vi "Thread@ElseIf__Parameter.vi"(1 "ParamterIn":string) -> (0 "ParamterOut":string)   [LabVIEW 2020]
panel:
  in  "Logic":string(combo)
  in  "Confirm":bool
  # "Thread@ElseIf $Logic"
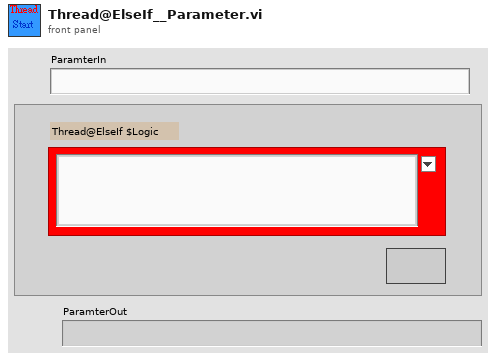
[diagram p1: front panel]
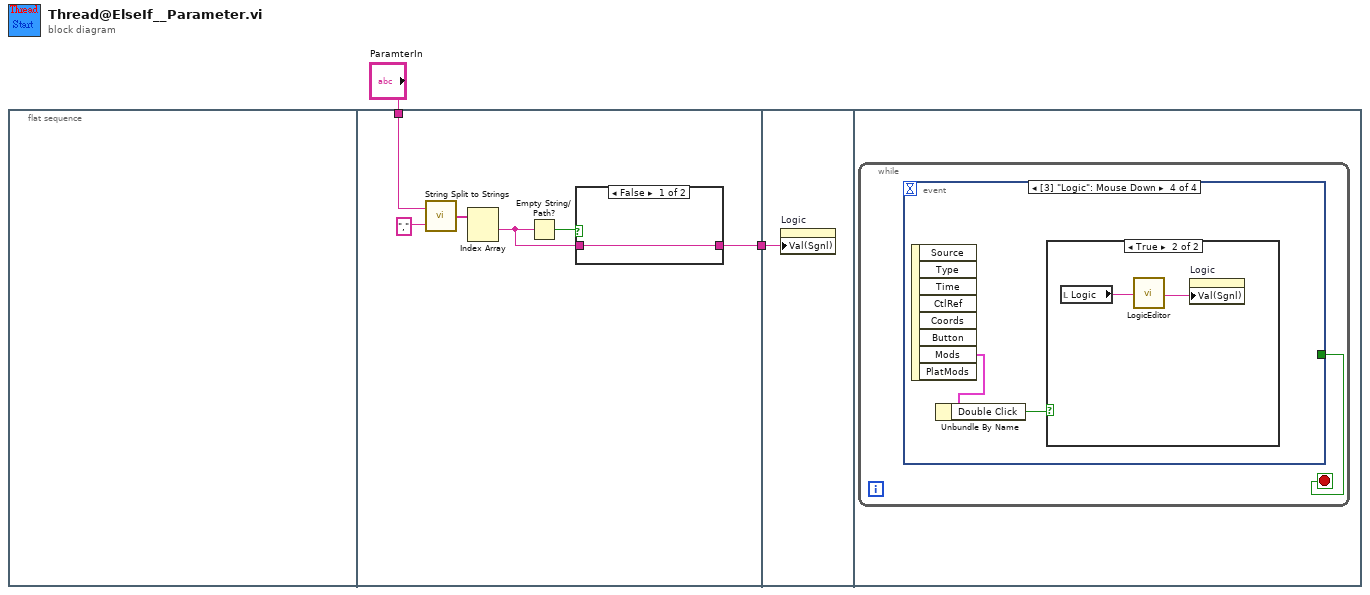
[diagram p0: block diagram]
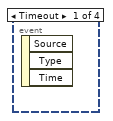
[diagram p3: hidden frame]
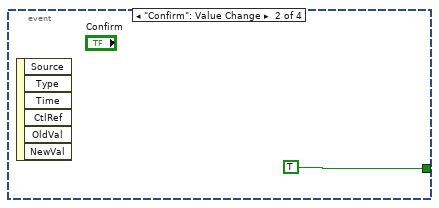
[diagram p4: hidden frame]
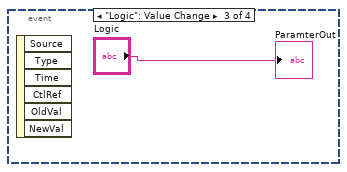
[diagram p5: hidden frame]
diagram:
  n1 = flat-sequence {
    tunnel: "ParamterIn" -> [w6]
    tunnel: [w3] -> w1
    tunnel: w1 -> [w10]
    frame #0 {
    }
    frame #1 {
      n2 = call "String Split to Strings.vi"("search string/char (-)"=",", "String"=w6) -> ("Array"=w8:string[])
      n3 = Index Array(array=w8) -> (element #1=w4:string)  [unwired: 2 in, 1 out]
      n4 = Empty String/Path?(string/path=w4) -> (empty?=w5:bool)
      n5 = case shown="False" w5 {
        tunnel: w4 -> [w9 _]
        tunnel: [w9 _] -> w3
        frame False {
        }
        frame True {
        }
      }
    }
    frame #2 {
      n6 = property on="Logic" class="CmbBox"("Val(Sgnl)"=w10) -> ()  [unwired: 2 in, 2 out]
    }
    frame #3 {
      n7 = while {
        stop <- w11 stop-if-true
        n8 = event shown="[3] \"Logic\": Mouse Down" {
          selector: _ -> [_ _ _ _]
          dyn-events: _ -> [_ _ _ _]
          timeout: _ -> [_ _ _ _]
          tunnel: [_ TRUE _ _] -> w11
          event Timeout {
            n9 = event-data() -> ()  [unwired: 1 in, 3 out]
          }
          event "Confirm": Value Change {
            n10 = event-data() -> ()  [unwired: 1 in, 6 out]
          }
          event "Logic": Value Change {
            n11 = event-data() -> ()  [unwired: 1 in, 6 out]
            "ParamterOut" <- "Logic"
          }
          event "Logic": Mouse Down {
            n12 = event-data() -> ("Mods"=w15:cluster{"Double Click":bool, "Menu Key":bool})  [unwired: 1 in, 7 out]
            n13 = Unbundle By Name(w15) -> ("Double Click"=w14:bool)
            n14 = case shown="True" w14 {
              frame False {
              }
              frame True {
                n15 = local read "Logic"() -> (w17:string)
                n16 = call "LogicEditor.vi"("Logic Express"=w17) -> ("LogicExpressOut"=w16:string)
                n17 = property on="Logic" class="CmbBox"("Val(Sgnl)"=w16) -> ()  [unwired: 2 in, 2 out]
              }
            }
          }
        }
      }
    }
  }
